vi "Object_Create.vi"(0 "reference in":refnum<class "Object.lvclass">, 1 "Object Attributes":T1, 5 "error in (no error)":errorcluster) -> (14 "reference out":refnum<class "Object.lvclass">, 19 "error out":errorcluster)   [LabVIEW 2014, in "Object.lvclass"]
uses:
  Object.lvclass
  Attributes.ctl
  Coordinates.ctl
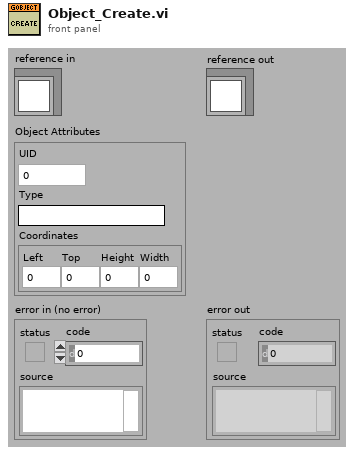
[diagram p1: front panel]
types:
  T1 = typedef "Object.lvclass/Attributes.ctl" = cluster{"UID":i32, "Type":string, "Coordinates":T2}
  T2 = typedef "Object.lvclass/Coordinates.ctl" = cluster{"Left":i32, "Top":i32, "Height":u32, "Width":u32}
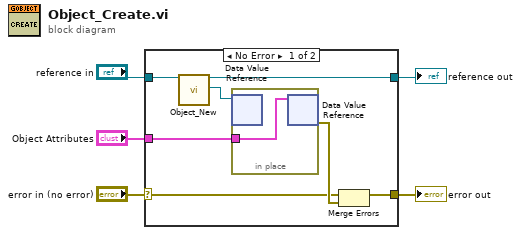
[diagram p0: block diagram]
diagram:
  n1 = case shown="No Error" "error in (no error)" {
    selector: "error in (no error)" -> [w6 w15]
    tunnel: [w9 w15] -> w4
    tunnel: "reference in" -> [w12 w14]
    tunnel: [w11 w14] -> w2
    tunnel: "Object Attributes" -> [w7 _]
    frame No Error {
      n2 = call "Object_New.vi"("reference in"=w12) -> ("reference out"=w11:refnum<class "Object.lvclass">, "DVRRefOut"=w8:refnum<data-value>)  [unwired: 15 in, 2 out]
      n3 = in-place {
        in-place-border: w7 -> [w13]
        n4 = in-place-dvr #1(w8) -> ()  [unwired: 2 out]
        n5 = in-place-dvr #1(w13) -> (w10:errorcluster)  [unwired: 1 out]
      }
      n6 = Merge Errors(w6, w10) -> (w9:errorcluster)
    }
    frame Error {
    }
  }
  "error out" <- w4
  "reference out" <- w2
